vi "Fit_Poly2Disc_fcn.vi"(3 "output control":T3, 4 "data":T4, 5 "X":dbl[](array[numeric])) -> (0 "error out":errorcluster, 1 "gradient":dbl[](array[numeric]), 2 "f(X)":dbl)   [LabVIEW 2012]
doc: "This template is the starting point for creating an objectivel function to be passed to the Unconstrained Optimization.vi."
uses:
  <vilib>/gmath/NumericalOptimization/objective function data.ctl
  <vilib>/Analysis/6fits.llb/General Linear Fit Algorithm.ctl
  <vilib>/Analysis/6fits.llb/Curve Fitting Criteria.ctl
  Displacement Data.ctl
  <vilib>/Analysis/polynomials.llb/Create Polynomial From Roots (DBL).vi
  <vilib>/Analysis/polynomials.llb/Polynomial Plot (Samples).vi
  <vilib>/Analysis/baseanly.llb/Mean (DBL).vi
  <vilib>/Analysis/NI_AALPro.lvlib
  <vilib>/Analysis/NI_AALBase.lvlib
  <vilib>/gmath/NI_Gmath.lvlib
panel:
  in  "Save?":bool
  in  "Picture Save Folder":path
  in  "Graph?":bool
  out "Displacement Graph":cluster{dbl[], "Best Polynomial Fit":dbl[]}[](graph)
  in  "method":T1 items=["Least Square", "Least Absolute Residual", "Bisquare"]
  in  "algorithm":T2 items=["SVD", "Givens", "Givens2", "Householder", "LU Decomposition", "Cholesky", "SVD for Rank Deficient H"]
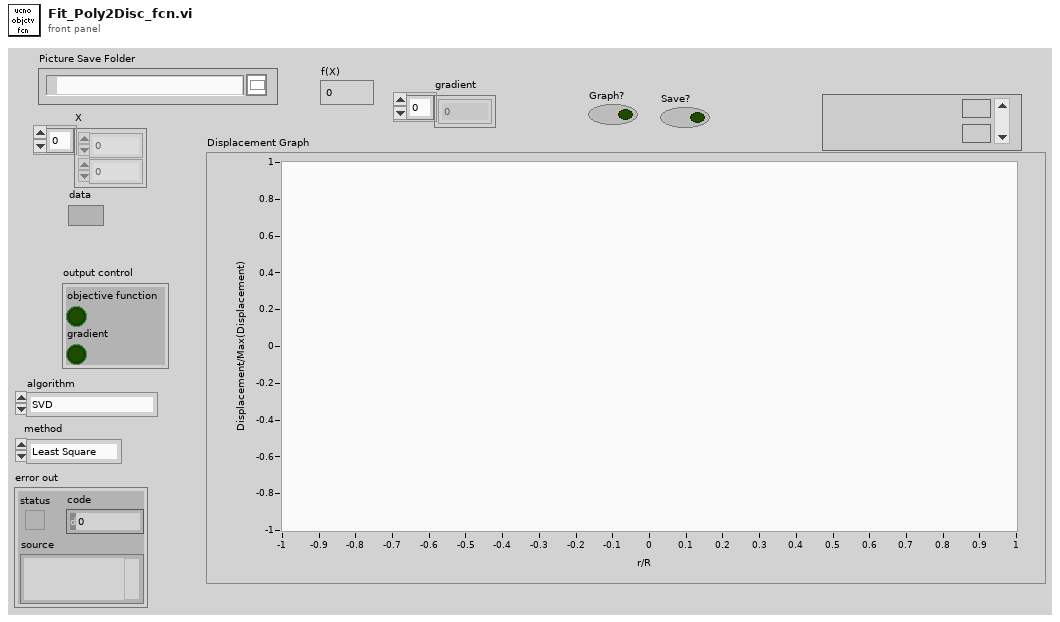
[diagram p1: front panel]
types:
  T1 = typedef "NI_AALPro.lvlib/Curve Fitting Criteria.ctl" = u16
  T2 = typedef "NI_AALPro.lvlib/General Linear Fit Algorithm.ctl" = u16
  T3 = cluster{"objective function":bool, "gradient":bool}
  T4 = typedef "NI_Gmath.lvlib/objective function data.ctl" = variant
  T5 = typedef "Displacement Data.ctl" = cluster{"Xd(t,r)":dbl[][], "Rc":dbl[]}
  T6 = typedef "imagedata.ctl" = cluster{"image type":i32, "image depth":i32, "image":u8[], "mask":u8[], "colors":u32[], "Rectangle":cluster{"left":i16, "top":i16, "right":i16, "bottom":i16}}
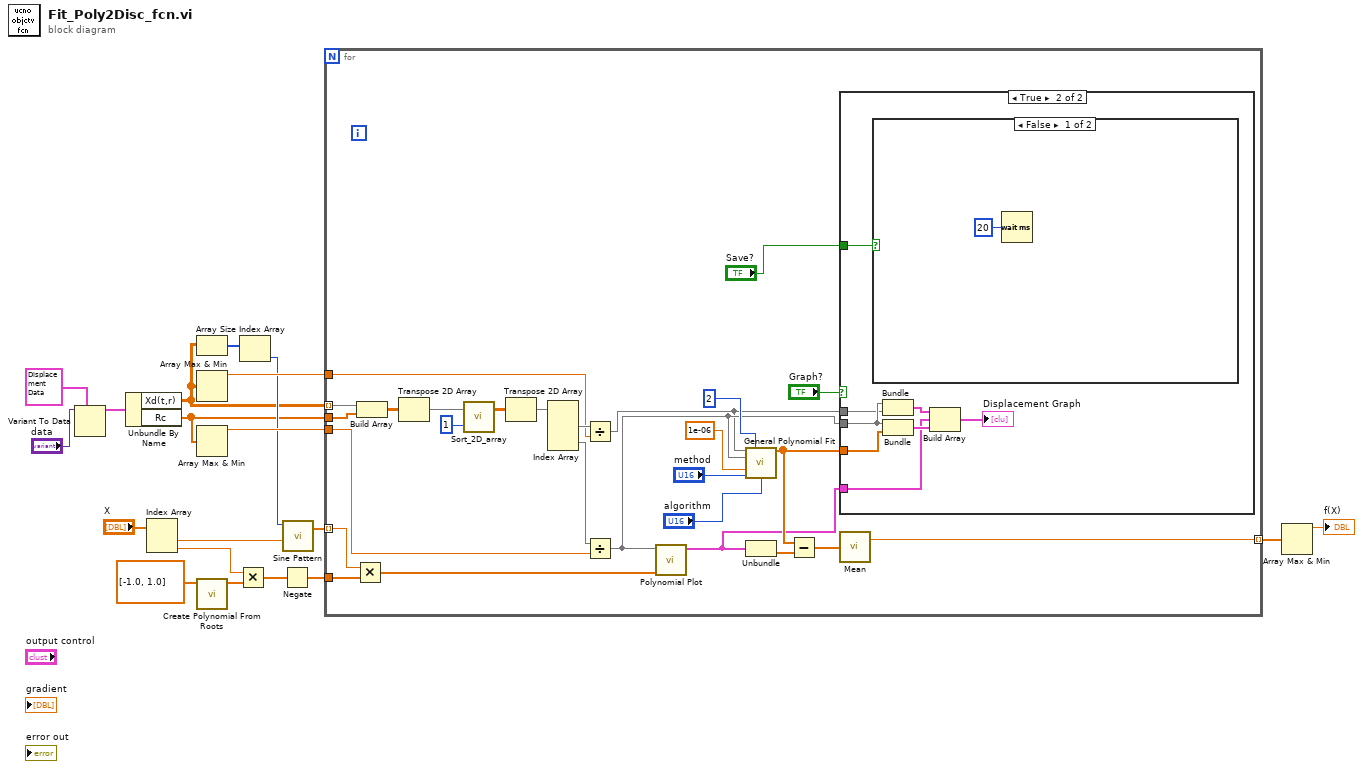
[diagram p0: block diagram]
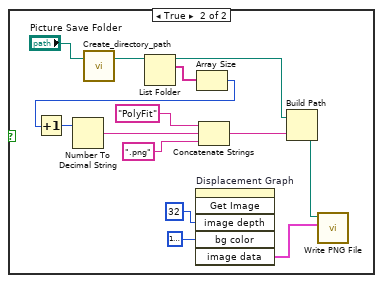
[diagram p3: hidden frame]
diagram:
  n1 = Variant To Data(type=T5 {"Xd(t,r)"=array25x40[1000 elements], "Rc"=[-10.5, -9.5, -8.5, -7.5, -6.5, -5.5, -4.5, -3.5, -2.5, -1.5, -19.5, -0.5, 0.5, 1.5, 2.5, 3.5, 4.5, 5.5, 6.5, 7.5, 8.5, -18.5, 9.5, 10.5, 11.5, 12.5, 13.5, 14.5, 15.5, 16.5, 17.5, 18.5, -17.5, 19.5, -16.5, -15.5, -14.5, -13.5, -12.5, -11.5]} ("Displacement Data"), Variant="data") -> (data=w4:T5)  [unwired: 1 in, 1 out]
  n2 = Unbundle By Name(w4) -> ("Xd(t,r)"=w3:dbl[][], "Rc"=w2:dbl[])
  n3 = Index Array(array="X") -> (element #1=w9:dbl, element #2=w1:dbl)  [unwired: 2 in]
  n4 = Array Size(array=w3) -> (size(s)=w15:i32[])
  n5 = Array Max & Min(array=w3) -> (max value=w18:dbl)  [unwired: 3 out]
  n6 = Array Max & Min(array=w2) -> (max value=w19:dbl)  [unwired: 3 out]
  n7 = call-poly <vilib>:"Create Polynomial From Roots.vi"("Roots"=dbl[] [-1.0, 1.0]) -> ("P(x)"=w16:dbl[])  [unwired: 9 in, 1 out]
  n8 = Multiply(x=w1, y=w16) -> (x*y=w7:dbl[])
  n9 = Index Array(array=w15) -> (element=w14:i32)  [unwired: 1 in]
  n10 = Negate(x=w7) -> (-x=w12:dbl[])
  n11 = call <vilib>:"Sine Pattern.vi"("phase(degrees)"=w9, "samples"=w14) -> ("Sinusoidal Pattern"=w13:dbl[])  [unwired: 2 in, 1 out]
  n12 = for {
    tunnel: w3 -> [w33] mode=indexing
    tunnel: w2 -> [w42]
    tunnel: w19 -> [w38]
    tunnel: w18 -> [w32]
    tunnel: w13 -> [w31] mode=indexing
    tunnel: w12 -> [w30]
    tunnel: [w26] -> w11 mode=indexing
    n13 = Multiply(x=w31, y=w30) -> (x*y=w29:dbl[])
    n14 = Build Array(w33, w42) -> (w41:dbl[][])
    n15 = Transpose 2D Array(2D array=w41) -> (transposed array=w44:dbl[][])
    n16 = call "Sort_2D_array.vi"("Column index to sort on"=1, "unsorted array"=w44) -> ("sorted array"=w45:dbl[][])  [unwired: 1 out]
    n17 = Transpose 2D Array(2D array=w45) -> (transposed array=w43:dbl[][])
    n18 = Index Array(array=w43) -> (element #1=w39:dbl[], element #2=w40:dbl[])  [unwired: 4 in]
    n19 = Divide(x=w39, y=w32) -> (x/y=w23:dbl[])
    n20 = Divide(x=w40, y=w38) -> (x/y=w24:dbl[])
    n21 = call-poly <vilib>:"Polynomial Plot.vi"("P(x)"=w29, "X"=w24) -> ("polynomial plot"=w22:cluster{dbl[], "P(A)":dbl[]})  [unwired: 8 in, 1 out]
    n22 = call <vilib>:"General Polynomial Fit.vi"("Y"=w23, "polynomial order"=2, "X"=w24, "tolerance"=1e-06, "method"="method", "algorithm"="algorithm") -> ("Best Polynomial Fit"=w25:dbl[])  [unwired: 6 in, 3 out]
    n23 = Unbundle(w22) -> ("P(A)"=w28:dbl[])  [unwired: 1 out]
    n24 = Subtract(x=w25, y=w28) -> (x-y=w27:dbl[])
    n25 = case shown="True" "Graph?" {
      tunnel: w25 -> [_ w54]
      tunnel: w24 -> [_ w53]
      tunnel: w23 -> [_ w52]
      tunnel: w22 -> [_ w48]
      tunnel: "Save?" -> [_ w47]
      frame False {
      }
      frame True {
        n26 = case shown="False" w47 {
          frame False {
            n27 = Wait (ms)(milliseconds to wait=u32 20) -> ()  [unwired: 1 out]
          }
          frame True {
            n28 = call "Create_directory_path.vi"("Path name"="Picture Save Folder") -> ("Path name Out"=w60:path)  [unwired: 1 in, 1 out]
            n29 = List Folder(path=w60) -> (path out=w59:path, filenames=w58:string[])  [unwired: 3 in, 2 out]
            n30 = invoke on="Displacement Graph" class="XYGraph (strict)" method="Get Image"("image depth"=32 ("Image Depth"), "bg color"=u32 16777216 ("Color")) -> ("image data"=w64:T6)  [unwired: 4 in, 5 out]
            n31 = Array Size(array=w58) -> (size(s)=w56:i32)
            n32 = Increment(x=w56) -> (x+1=w57:i32)
            n33 = Number To Decimal String(number=w57) -> (decimal integer string=w69:string)  [unwired: 1 in]
            n34 = Concatenate Strings("PolyFit" ("string"), w69, ".png" ("string")) -> (w66:string)
            n35 = Build Path(base path=w59, name or relative path=w66) -> (appended path=w65:path)
            n36 = call <vilib>:"Write PNG File.vi"("image data"=w64, "path to PNG file"=w65) -> ()  [unwired: 8 in, 2 out]
          }
        }
        n37 = Bundle(w53, w52) -> (w51:cluster{dbl[], dbl[]})  [unwired: 1 in]
        n38 = Bundle(w53, "Best Polynomial Fit"=w54) -> (w49:cluster{dbl[], "Best Polynomial Fit":dbl[]})  [unwired: 1 in]
        n39 = Build Array(w51, w48, w49) -> (→"Displacement Graph":cluster{dbl[], "Best Polynomial Fit":dbl[]}[])
      }
    }
    n40 = call-poly <vilib>:"Mean.vi"("X"=w27) -> ("mean"=w26:dbl)  [unwired: 1 out]
  }
  n41 = Array Max & Min(array=w11) -> (max value=→"f(X)":dbl)  [unwired: 3 out]
